vi "setFPGA.vi"(10 "FPGA":refnum<class "FPGA.lvclass">, 11 "HealthAndStatusControlFIFO in":refnum<class "HealthAndStatusControlFIFO.lvclass">) -> (3 "HealthAndStatusControlFIFO out":refnum<class "HealthAndStatusControlFIFO.lvclass">)   [LabVIEW 2016, in "HealthAndStatusControlFIFO.lvclass"]
uses:
  HealthAndStatusControlFIFO.lvclass
  FPGA/FPGA.lvclass
  HealthAndStatusControlFIFO.lvclass/HealthAndStatusControlFIFO.ctl
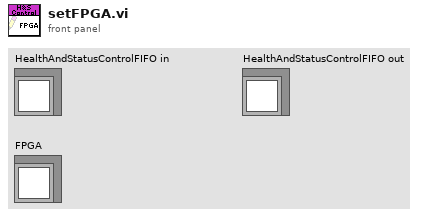
[diagram p1: front panel]
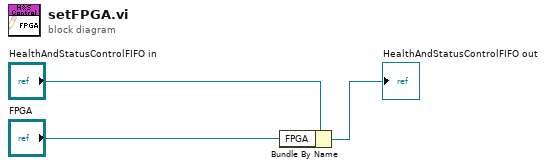
[diagram p0: block diagram]
diagram:
  n1 = Bundle By Name(cluster="HealthAndStatusControlFIFO in", "FPGA"="FPGA") -> (→"HealthAndStatusControlFIFO out":refnum<class "HealthAndStatusControlFIFO.lvclass">)
